vi "merFISH_read_valve_number.vi"(4 "error in":errorcluster, 5 "Probe #":i32, 6 "ProbeList Refnum":refnum<vi>, 7 "Valve # IN":i32) -> (0 "error out":errorcluster, 1 "Valve # OUT":i32)   [LabVIEW 2015]
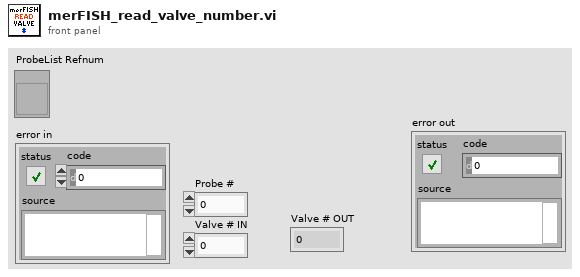
[diagram p1: front panel]
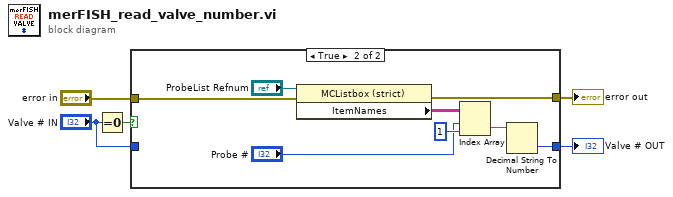
[diagram p0: block diagram]
diagram:
  n1 = Equal To 0?(x="Valve # IN") -> (x = 0?=w5:bool)
  n2 = case shown="True" w5 {
    tunnel: [w7 w10] -> w3
    tunnel: "Valve # IN" -> [w7 _]
    tunnel: "error in" -> [w6 w9]
    tunnel: [w6 w8] -> w1
    frame False {
    }
    frame True {
      n3 = property class="MCListbox (strict)"(reference="ProbeList Refnum", error in=w9) -> (error out=w8:errorcluster, "ItemNames"=w14:string[][])  [unwired: 1 out]
      n4 = Index Array(array=w14, index (row)="Probe #", index (col)=1 ("disabled index (col)")) -> (element=w11:string)
      n5 = Decimal String To Number(string=w11) -> (number=w10:i32)  [unwired: 2 in, 1 out]
    }
  }
  "Valve # OUT" <- w3
  "error out" <- w1
